vi "SubVI Tester.vi"() -> ()   [LabVIEW 2025]
panel:
  out "standard warning":string
  out "Warning?":bool
  in  "Cluster":T1
  in  "Min Temperature":dbl=10.0
  in  "Max Temperature":dbl=30.0
  in  "Stop":bool
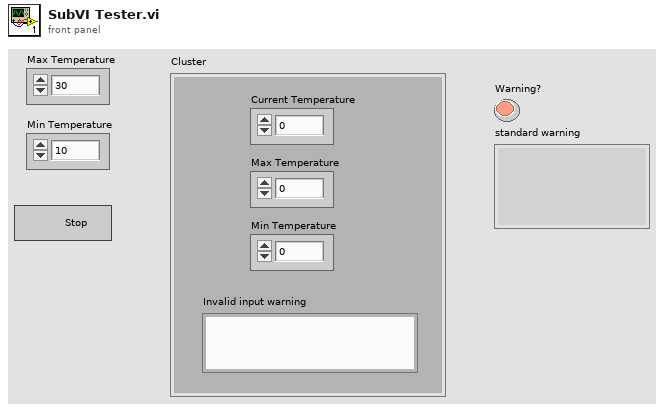
[diagram p1: front panel]
types:
  T1 = cluster{"Current Temperature":dbl, "Max Temperature":dbl, "Min Temperature":dbl, "Invalid input warning":string}
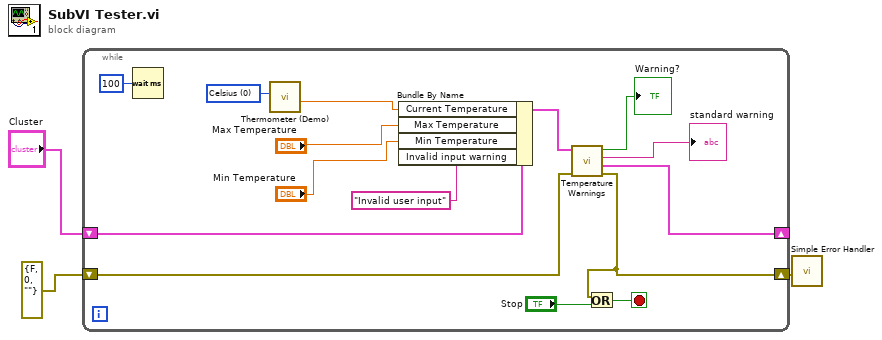
[diagram p0: block diagram]
diagram:
  n1 = while {
    shift-right: [w8] -> w3
    shift-left: errorcluster {"status"=FALSE, "code"=0, "source"=""} ("error in") -> [w9]
    shift-right: [w7] -> _
    shift-left: "Cluster" -> [w15]
    stop <- w16 stop-if-true
    w4 = u16 0 items=["Celsius", "Fahrenheit"] ("Units (0: Celsius)")
    n2 = Wait (ms)(milliseconds to wait=u32 100) -> ()  [unwired: 1 out]
    n3 = call "Thermometer (Demo).vi"("Units (0: Celsius)"=w4) -> ("Temperature Value"=w14:dbl)  [unwired: 10 in]
    n4 = Bundle By Name(cluster=w15, "Current Temperature"=w14, "Max Temperature"="Max Temperature", "Min Temperature"="Min Temperature", "Invalid input warning"="Invalid user input") -> (w10:T1)
    n5 = call "Temperature Warnings.vi"("Error In"=w9, "Cluster"=w10) -> ("Error Out"=w8:errorcluster, "Cluster 2"=w7:T1, "standard warning"=→"standard warning":string, "Warning?"=→"Warning?":bool)  [unwired: 6 in]
    n6 = Or(x=w8, y="Stop") -> (x .or. y?=w16:bool)
  }
  n7 = call <vilib>:"Simple Error Handler.vi"("error in (no error)"=w3) -> ()  [unwired: 4 in, 5 out]
